vi "YAML Get Field Value.vi"(10 "field name":string, 11 "array of strings":string[][](array[string])) -> (3 "field value":string)   [LabVIEW 2011]
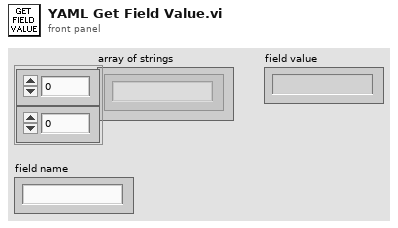
[diagram p1: front panel]
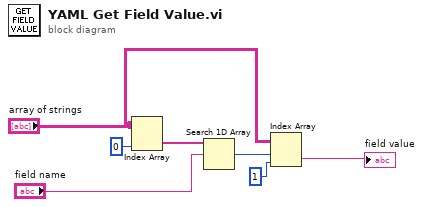
[diagram p0: block diagram]
diagram:
  n1 = Index Array(array="array of strings", index (col)=0 ("disabled index (col)")) -> (element=w2:string[])  [unwired: 1 in]
  n2 = Search 1D Array(1D array=w2, element="field name") -> (index of element=w1:i32)  [unwired: 1 in]
  n3 = Index Array(array="array of strings", index (row)=w1, index (col)=1 ("disabled index (col)")) -> (element=→"field value":string)
